vi "Write Events.vi"(8 "error in (no error)":errorcluster, 10 "Events":T1, 11 "Laser State Data in":refnum<class "Laser State Data.lvclass">) -> (0 "error out":errorcluster, 3 "Laser State Data out":refnum<class "Laser State Data.lvclass">)   [LabVIEW 2022 SP3, in "Laser State Data.lvclass"]
uses:
  Laser State Data.lvclass
  Laser State Data.lvclass/Laser State Data.ctl
  Laser State.ctl
  Events.ctl
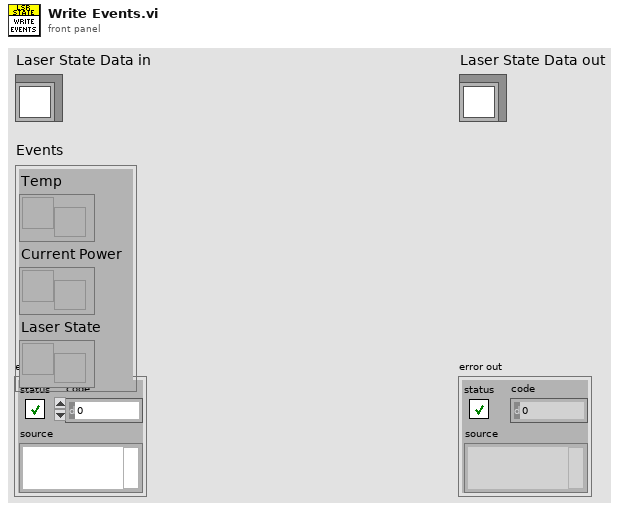
[diagram p1: front panel]
types:
  T1 = typedef "Laser State Data.lvclass/Events.ctl" = cluster{"Temp":refnum<user-event>, "Current Power":refnum<user-event>, "Laser State":refnum<user-event>}
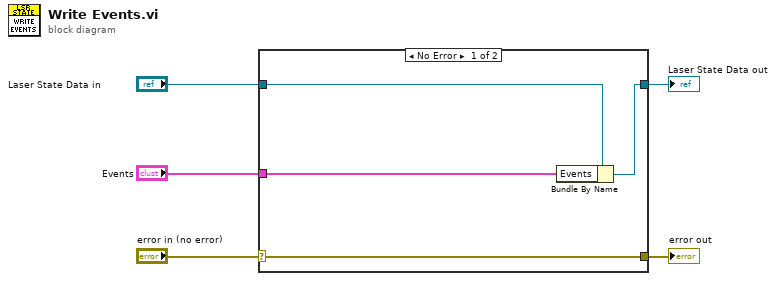
[diagram p0: block diagram]
diagram:
  n1 = case shown="No Error" "error in (no error)" {
    selector: "error in (no error)" -> [w9 w10]
    tunnel: [w9 w10] -> w4
    tunnel: [w7 w11] -> w2
    tunnel: "Laser State Data in" -> [w8 w11]
    tunnel: "Events" -> [w6 _]
    frame No Error {
      n2 = Bundle By Name(cluster=w8, "Events"=w6) -> (w7:refnum<class "Laser State Data.lvclass">)
    }
    frame Error {
    }
  }
  "error out" <- w4
  "Laser State Data out" <- w2
